vi "Draw Mic.vi"(0 "picture in":picture, 5 "center":cluster{"X":i32, "Y":i32}, 7 "Width":i32=3, 9 "Index":i32, 11 "Selected":bool) -> (4 "picture out":picture)   [LabVIEW 2015, in "HRTF Config.xctl"]
uses:
  HRTF Config.xctl
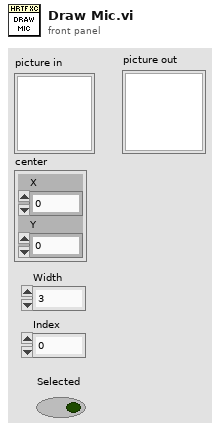
[diagram p1: front panel]
types:
  T1 = cluster{"left":i16, "top":i16, "right":i16, "bottom":i16}
  T2 = cluster{"left":i32, "top":i32, "right":i32, "bottom":i32}
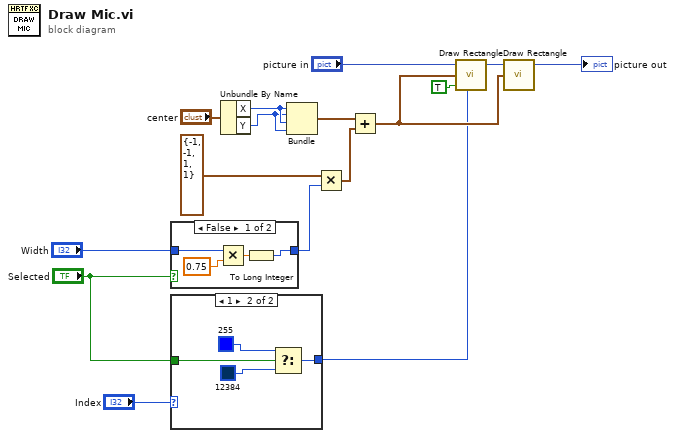
[diagram p0: block diagram]
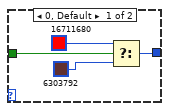
[diagram p3: hidden frame]
diagram:
  n1 = case shown="False" "Selected" {
    tunnel: [w17 w21] -> w2
    tunnel: "Width" -> [w20 w21]
    frame False {
      n2 = Multiply(x=w20, y=0.75) -> (x*y=w18:dbl)
      n3 = To Long Integer(number=w18) -> (32bit integer=w17:i32)
    }
    frame True {
    }
  }
  n4 = case shown="1" "Index" {
    tunnel: "Selected" -> [w24 w28]
    tunnel: [w22 w26] -> w4
    frame 0, Default {
      n5 = Select(t=u32 16711680, s=w24, f=u32 6303792) -> (s? t:f=w22:u32)
    }
    frame 1 {
      n6 = Select(t=u32 255, s=w28, f=u32 12384) -> (s? t:f=w26:u32)
    }
  }
  n7 = Unbundle By Name("center") -> ("X"=w11:i32, "Y"=w10:i32)
  n8 = Bundle("X"=w11, "Y"=w10, "X"=w11, "Y"=w10) -> (w13:cluster{"X":i32, "Y":i32, "X":i32, "Y":i32})  [unwired: 1 in]
  n9 = Multiply(x=T1 {"left"=-1, "top"=-1, "right"=1, "bottom"=1} ("rect"), y=w2) -> (x*y=w14:T2)
  n10 = Add(x=w13, y=w14) -> (x+y=w7:cluster{i32, i32, i32, i32})
  n11 = call <vilib>:"Draw Rectangle.vi"("picture"="picture in", "rect"=w7, "fill?(F)"=TRUE, "color(black)"=w4) -> ("new picture"=w8:picture)  [unwired: 5 in]
  n12 = call <vilib>:"Draw Rectangle.vi"("picture"=w8, "rect"=w7) -> ("new picture"=→"picture out":picture)  [unwired: 7 in]
